vi "ULS Basic Tags.vi"(5 "Scan Rate(sample/sec)":dbl=1000.0 format="%#_13g", 7 "Objective":u32=1, 8 "error in (no error)":errorcluster, 9 "Scan Dimension":T1={"ROI"=enum."Rectangle", "Z layer count"=255, "Time Lapse"=enum."None"}, 10 "Scanner Component":T2={"Detector"=enum."Andor CCD", "Mover"=enum."None"}, 11 "IFD in":refnum<class "IFD.lvclass">) -> (0 "error out":errorcluster, 3 "IFD out":refnum<class "IFD.lvclass">)   [LabVIEW 2016, in "IFD.lvclass"]
uses:
  IFD.lvclass
  Tag/IFD_Tag.lvclass/IFD_Tag.ctl
  IFD.lvclass/IFD.ctl
  Tag/IFD_Tag.lvclass
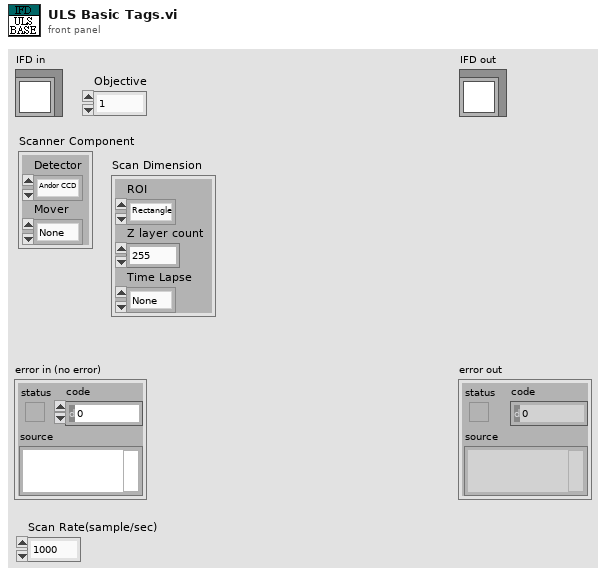
[diagram p1: front panel]
types:
  T1 = cluster{"ROI":enum8{"Undefined: No Ref", "Point", "Line", "Rectangle", "Square"}, "Z layer count":u8, "Time Lapse":enum8{"None", "Toe to Head", "Head to Head"}}
  T2 = cluster{"Detector":enum16{"Mightex BUF CCD", "PMT", "Andor CCD"}, "Mover":enum16{"None", "Galvo", "Sigmakoki Stage"}}
  T3 = enum16{"Undefined(DO NOT USE)", "U8", "ASCII", "U16", "U32", "RATIONAL", "I8", "Undefined 8 bit", "I16", "I32", "SRATIONAL", "SGL", "DBL"}
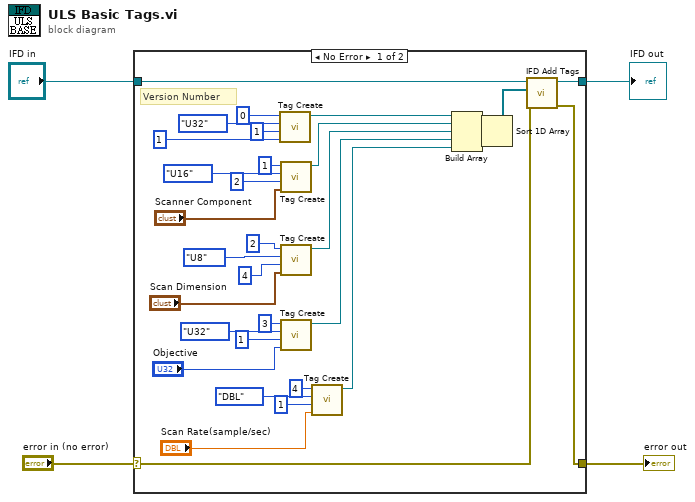
[diagram p0: block diagram]
diagram:
  n1 = case shown="No Error" "error in (no error)" {
    selector: "error in (no error)" -> [w19 w37]
    tunnel: [w18 w37] -> w3
    tunnel: [w34 w36] -> w1
    tunnel: "IFD in" -> [w35 w36]
    frame No Error {
      # "Version Number"
      n2 = call "Tag Create.vi"("Data"=u32 1, "Data Count"=u32 1, "Data Type"=T3."U32", "Tag ID"=u16 0) -> ("IFD_Tag out"=w25:refnum<class "IFD_Tag.lvclass">)  [unwired: 7 in]
      n3 = call "Tag Create.vi"("Data"="Scanner Component", "Data Count"=u32 2, "Data Type"=T3."U16", "Tag ID"=u16 1) -> ("IFD_Tag out"=w24:refnum<class "IFD_Tag.lvclass">)  [unwired: 7 in]
      n4 = call "Tag Create.vi"("Data"="Scan Dimension", "Data Count"=u32 4, "Data Type"=T3."U8", "Tag ID"=u16 2) -> ("IFD_Tag out"=w23:refnum<class "IFD_Tag.lvclass">)  [unwired: 7 in]
      n5 = call "Tag Create.vi"("Data"="Objective", "Data Count"=u32 1, "Data Type"=T3."U32", "Tag ID"=u16 3) -> ("IFD_Tag out"=w22:refnum<class "IFD_Tag.lvclass">)  [unwired: 7 in]
      n6 = call "Tag Create.vi"("Data"="Scan Rate(sample/sec)", "Data Count"=u32 1, "Data Type"=T3."DBL", "Tag ID"=u16 4) -> ("IFD_Tag out"=w21:refnum<class "IFD_Tag.lvclass">)  [unwired: 7 in]
      n7 = Build Array(w25, w24, w23, w22, w21) -> (w20:refnum<class "IFD_Tag.lvclass">[])
      n8 = Sort 1D Array(array=w20) -> (sorted array=w5:refnum<class "IFD_Tag.lvclass">[])
      n9 = call "IFD Add Tags.vi"("error in (no error)"=w19, "Tag(s)"=w5, "IFD in"=w35) -> ("error out"=w18:errorcluster, "IFD out"=w34:refnum<class "IFD.lvclass">)  [unwired: 7 in]
    }
    frame Error {
    }
  }
  "error out" <- w3
  "IFD out" <- w1
